vi "Convert rate.vi"(10 "DDC IQ rates (kHz)":dbl[](array[numeric])) -> (2 "ddc.out.rate":fxp<+,48,1>[](array[numeric]) format="%.48g")   [LabVIEW 2015, in "7976R_v1.lvclass"]
uses:
  <userlib>/SE-APP-Receiver/NI5772/7976R_v1/7976R_v1.lvclass
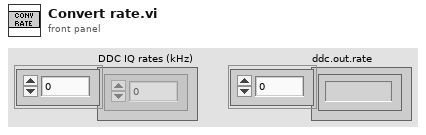
[diagram p1: front panel]
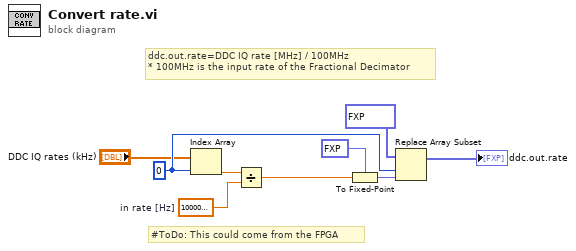
[diagram p0: block diagram]
diagram:
  w7 = 0 ("index")
  w3 = 100000000.0  # in rate [Hz]
  # "#ToDo: This could come from the FPGA"
  # "ddc.out.rate=DDC IQ rate [MHz] / 100MHz\n* 100MHz is the input rate of the Fractional Decimator"
  n1 = Index Array(array="DDC IQ rates (kHz)", index=w7) -> (element=w2:dbl)
  n2 = Divide(x=w2, y=w3) -> (x/y=w4:dbl)
  n3 = To Fixed-Point(fixed-point type=fxp<+,48,1> 0.0 ("ddc.0.output.sample.rate"), number=w4) -> (fixed-point=w8:fxp<+,48,1>)
  n4 = Replace Array Subset(array=fxp<+,48,1>[] [1.999999999999993, 0.0, 0.0, 0.0, 0.0, 0.0, 0.0, 0.0, 0.0, 0.0, 0.0, 0.0, 0.0, 0.0, 0.0, 0.0] ("ddc.out.rate"), new element=w8, index=w7) -> (→"ddc.out.rate":fxp<+,48,1>[])
